vi "Set Frequency Line.vi"(8 "error in (no error)":errorcluster {"code" format="%.0x"}, 9 "Position":dbl, 10 "Index":i32=1 format="%.0g", 11 "instrument handle":refnum<k15>) -> (0 "error out":errorcluster {"code" format="%.0x"}, 3 "instrument handle out":refnum<k15>)   [LabVIEW 2009, in "Keysight XSAn.lvlib"]
doc: "Selects the Frequency Line control.\n\nSupported Models: M9290A, M9410A, N8973B, N8974B, N8975B, N8976B, N9000A, N9000B, N9010A, N9010B, N9020A, N9020B, N9030A, N9030B, N9038A, N9040B, N9041B, SPN9003A, SPN9026A."
uses:
  <instrlib>/Keysight XSAn/Keysight XSAn.lvlib
  AgXSAn.dll
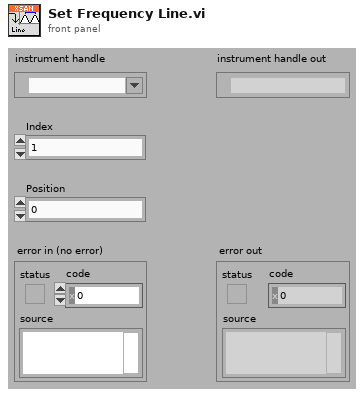
[diagram p1: front panel]
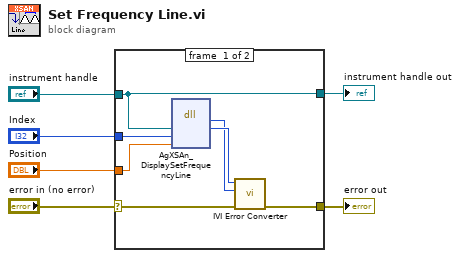
[diagram p0: block diagram]
diagram:
  n1 = case shown="No Error" "error in (no error)" {
    selector: "error in (no error)" -> [w11 w15]
    tunnel: [w10 w15] -> w6
    tunnel: "instrument handle" -> [w7 w14]
    tunnel: "Index" -> [w9 _]
    tunnel: "Position" -> [w8 _]
    tunnel: [w7 w14] -> w1
    frame #0 {
      n2 = dll-call lib="AgXSAn**.dll" fn="AgXSAn_DisplaySetFrequencyLine"("Vi"=w7, "Index"=w9, "Position"=w8) -> (w12:i32, "Vi"=w13:u32)  [unwired: 5 in, 2 out]
      n3 = call <instrlib>:"IVI Error Converter.vi"("error in (no error)"=w11, "IVI error code (0)"=w12, "instrument handle"=w13) -> ("error out"=w10:errorcluster)  [unwired: 7 in, 1 out]
    }
    frame #1 {
    }
  }
  "error out" <- w6
  "instrument handle out" <- w1
